vi "Startup 1.vi"(6 "LabVIEW Web Service":refnum<class "Web Service.lvclass">) -> ()   [LabVIEW 2014]
uses:
  <vilib>/wsapi/Web Service.lvclass
  DataManager/StateStore/Controls/DataFunction.ctl
panel:
  out "Array":cluster{"uuid":string, "int":i32}[](array[cluster])
  # "Use the web service input terminal to call the VIs on the Service subpalette of the Web Services palette. Do not remove it from the connector pane unless you don't need access to the palette."
  # "Any additional terminals added to the connector pane of a startup VI will be ignored."
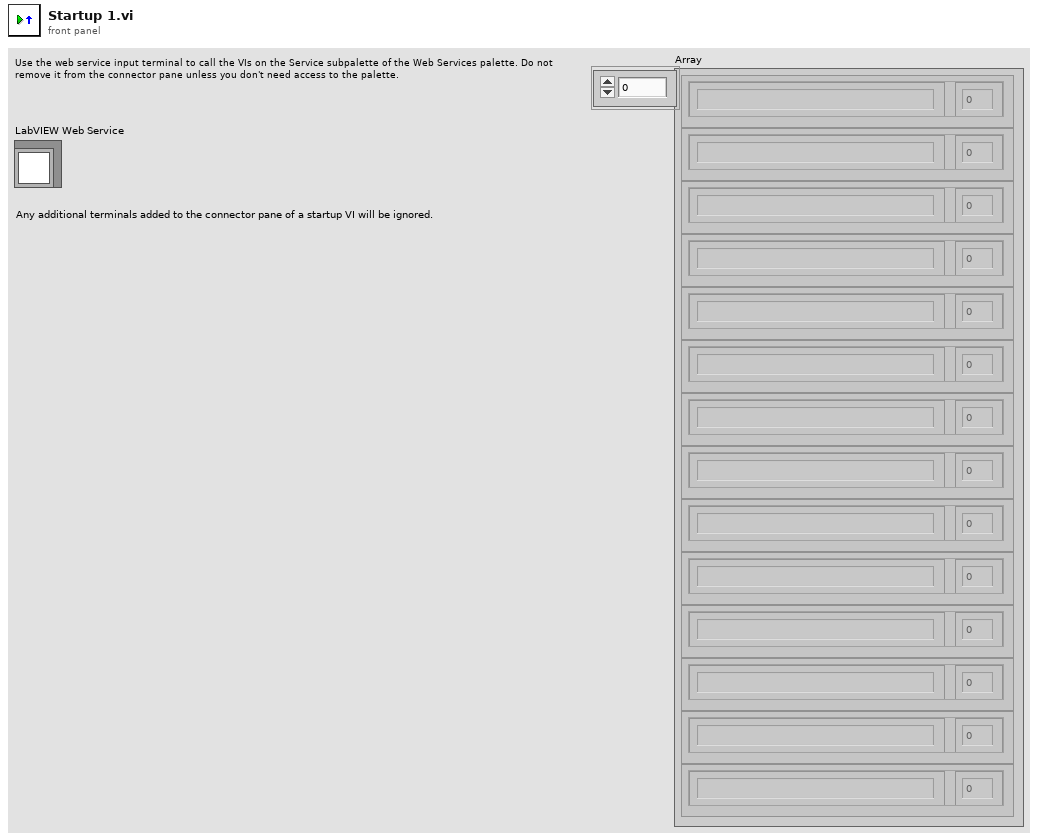
[diagram p1: front panel]
types:
  T1 = typedef "DataFunction.ctl" = enum16{"Initialise", "Release", "Get Data", "Set Data", "Preview Data"}
  T2 = typedef "CData Core Control.ctl" = cluster{"train_data_array":cluster{"uuid":string, "int":i32, "posit_array":cluster{"x":dbl, "y":dbl, "z":dbl}[]}[], "train_control_array":cluster{"uuid":string, "throttle":dbl, "brake":dbl, "horn":dbl, "wait":dbl, "name":string, "mode":string, "dest":string}[], "switch_data_array":cluster{"switch_posit":cluster{"x":dbl, "y":dbl, "z":dbl}, "manual":bool}[], "switch_control_array":cluster{"switch_posit":cluster{"x":dbl, "y":dbl, "z":dbl}, "switch":bool, "invert":bool, "wait":dbl}[]}
  T3 = cluster{"uuid":string, "int":i32, "posit_array":cluster{"x":dbl, "y":dbl, "z":dbl}[]}[]
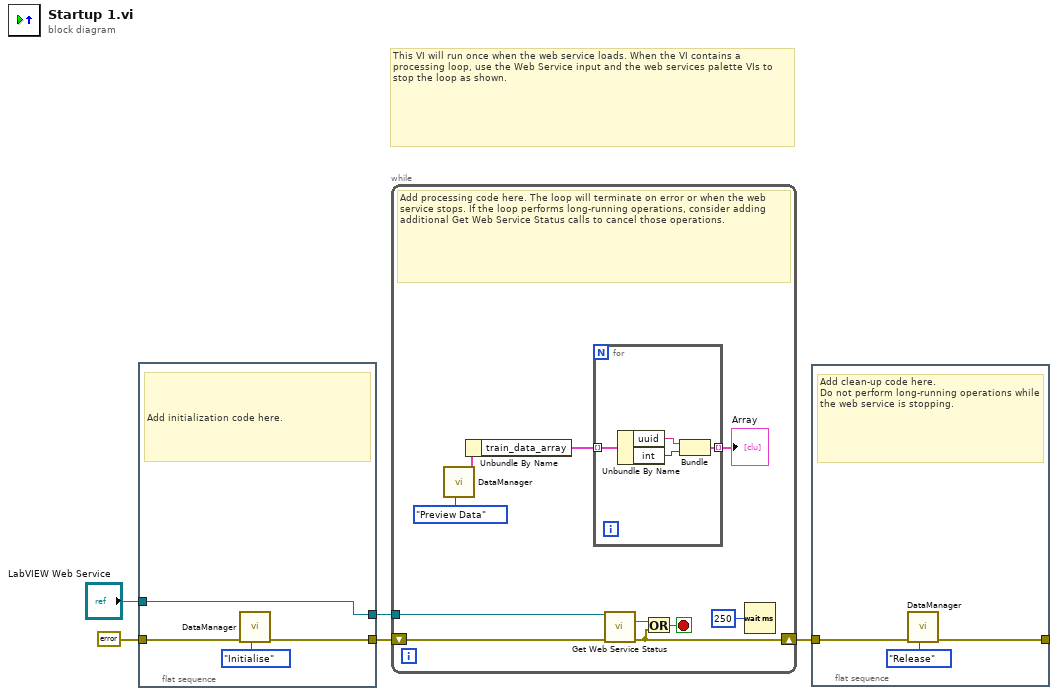
[diagram p0: block diagram]
diagram:
  # "This VI will run once when the web service loads. When the VI contains a processing loop, use the Web Service input and the web services palette VIs to stop the loop as shown."
  n1 = flat-sequence {
    tunnel: "LabVIEW Web Service" -> [w9]
    tunnel: [w9] -> w4
    tunnel: [w7] -> w3
    tunnel: errorcluster {"status"=FALSE, "code"=0, "source"=""} ("error constant") -> [w8]
    frame #0 {
      # "Add initialization code here."
      n2 = call "DataManager.vi"("DataFunction"=DataFunction."Initialise", "error in (no error)"=w8) -> ("error out"=w7:errorcluster)  [unwired: 8 in, 1 out]
    }
  }
  n3 = while {
    tunnel: w4 -> [w18]
    shift-right: [w15] -> w1
    shift-left: w3 -> [w16]
    stop <- w17 stop-if-true
    # "Add processing code here. The loop will terminate on error or when the web service stops. If the loop performs long-running operations, consider adding additional Get Web Service Status calls to cancel those operations."
    n4 = call "DataManager.vi"("DataFunction"=DataFunction."Preview Data") -> ("CData Out"=w12:T2)  [unwired: 9 in, 1 out]
    n5 = Unbundle By Name(w12) -> ("train_data_array"=w11:T3)
    n6 = for {
      tunnel: w11 -> [w23] mode=indexing
      tunnel: [w20] -> w10 mode=indexing
      n7 = Unbundle By Name(w23) -> ("uuid"=w21:string, "int"=w22:i32)
      n8 = Bundle("uuid"=w21, "int"=w22) -> (w20:cluster{"uuid":string, "int":i32})  [unwired: 1 in]
    }
    "Array" <- w10
    n9 = call <vilib>:"Get Web Service Status.vi"("LabVIEW Web Service"=w18, "error in (no error)"=w16) -> ("service stopping?"=w19:bool, "error out"=w15:errorcluster)  [unwired: 11 in, 1 out]
    n10 = Or(x=w19, y=w15) -> (x .or. y?=w17:bool)
    n11 = Wait (ms)(milliseconds to wait=u32 250) -> ()  [unwired: 1 out]
  }
  n12 = flat-sequence {
    tunnel: w1 -> [w25]
    tunnel: [w24] -> _
    frame #0 {
      # "Add clean-up code here.\nDo not perform long-running operations while the web service is stopping."
      n13 = call "DataManager.vi"("DataFunction"=DataFunction."Release", "error in (no error)"=w25) -> ("error out"=w24:errorcluster)  [unwired: 8 in, 1 out]
    }
  }
